vi "write resource name.vi"(8 "error in":errorcluster, 10 "resource name":string, 11 "Chassis in":refnum<class "Chassis.lvclass">) -> (0 "error out":errorcluster, 3 "Chassis out":refnum<class "Chassis.lvclass">)   [LabVIEW 2016, in "SMI.lvlib" / "Chassis.lvclass"]
uses:
  Chassis.lvclass
  Chassis.lvclass/Chassis.ctl
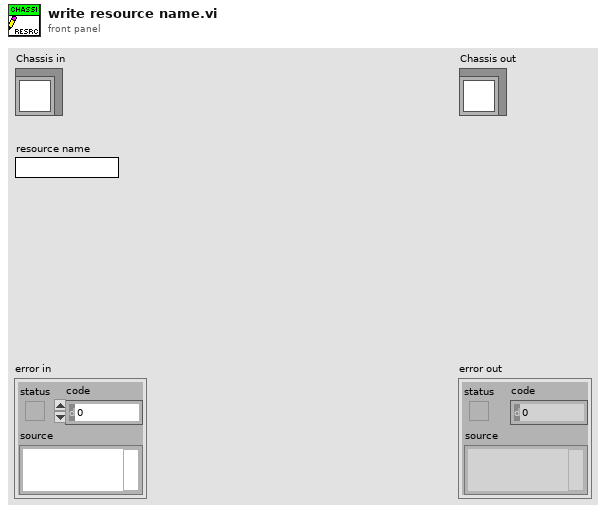
[diagram p1: front panel]
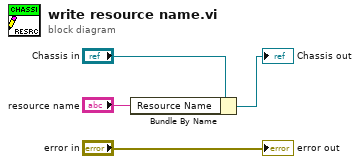
[diagram p0: block diagram]
diagram:
  n1 = Bundle By Name(cluster="Chassis in", "Resource Name"="resource name") -> (→"Chassis out":refnum<class "Chassis.lvclass">)
  "error out" <- "error in"
